vi "Publish.vi"(4 "ArgumentsKw":string, 6 "Arguments":string, 7 "Options":string, 8 "Error in":errorcluster, 9 "Time out (1000 ms)":i32=1000, 10 "Topic":string, 11 "WAMP Client in":refnum<class "WAMP Client.lvclass">) -> (0 "Error out":errorcluster, 3 "WAMP Client out":refnum<class "WAMP Client.lvclass">, 5 "WAMP Error":T1={"Details"="{}", "ArgumentKw Payload"="{}", "Error?"=FALSE, "Error URI"="", "Arguments Payload"=""})   [LabVIEW 2020, in "wamplv.lvlib" / "WAMP Client.lvclass"]
uses:
  WAMP Client.lvclass
  WAMP Client.lvclass/WAMP Client.ctl
  5e405bcd-0c6d-46be-a87b-06ec174a83c2.vi
  TypeDefs/WAMP error.ctl
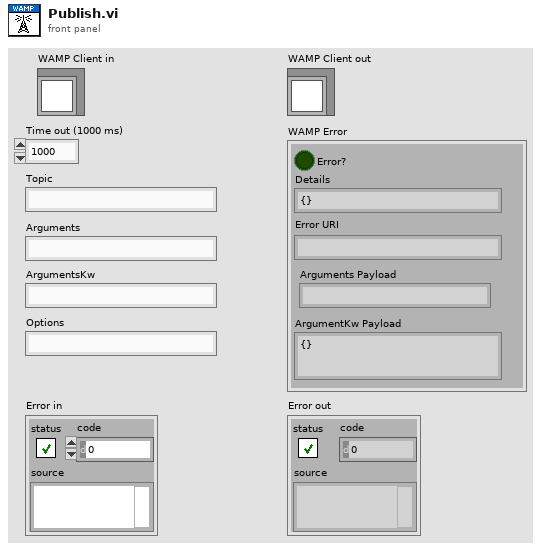
[diagram p1: front panel]
types:
  T1 = typedef "wamplv.lvlib/WAMP Client.lvclass/WAMP error.ctl" = cluster{"Details":string, "ArgumentKw Payload":string, "Error?":bool, "Error URI":string, "Arguments Payload":string}
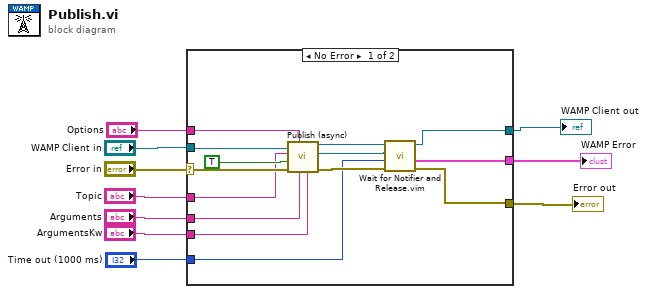
[diagram p0: block diagram]
diagram:
  n1 = case shown="No Error" "Error in" {
    selector: "Error in" -> [w23 w26]
    tunnel: [w20 w26] -> w9
    tunnel: [w11 w25] -> w7
    tunnel: "WAMP Client in" -> [w24 w25]
    tunnel: "Topic" -> [w15 _]
    tunnel: "Arguments" -> [w21 _]
    tunnel: "ArgumentsKw" -> [w22 _]
    tunnel: "Time out (1000 ms)" -> [w18 _]
    tunnel: [w17 _] -> w2
    tunnel: "Options" -> [w14 _]
    frame No Error {
      n2 = call "Publish (async).vi"("ArgumentsKw"=w22, "Arguments"=w21, "Options"=w14, "Error in"=w23, "Notify result"=TRUE ("Request Ack."), "Topic"=w15, "WAMP Client in"=w24) -> ("Error cout"=w19:errorcluster, "notifier out"=w13:refnum<notifier>, "WAMP Client out"=w12:refnum<class "WAMP Client.lvclass">)  [unwired: 2 in]
      n3 = call "Wait for Notifier and Release.vim"("error in (no error)"=w19, "timeout in ms (0)"=w18, "Notifier in"=w13, "WAMP Client in"=w12) -> ("error out"=w20:errorcluster, "WAMP Error"=w17:T1, "WAMP Client out"=w11:refnum<class "WAMP Client.lvclass">)  [unwired: 4 in, 1 out]
    }
    frame Error {
    }
  }
  "Error out" <- w9
  "WAMP Client out" <- w7
  "WAMP Error" <- w2
